vi "Add Bus Received Frames.vi"   [LabVIEW 2019, in "XNET-Bus-Load-Calculator.lvlib"]
uses:
  XNET-Bus-Load-Calculator.lvlib
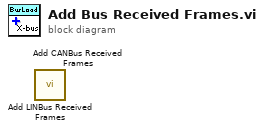
[diagram p0: block diagram]
diagram:
  n1 = call "Add LINBus Received Frames.vi"() -> ()  [unwired: 10 in, 2 out]
  n2 = call "Add CANBus Received Frames.vi"() -> ()  [unwired: 10 in, 2 out]
